vi "receiveBLMessages.vi"(8 "Error in":errorcluster {"code" format="%.0x"}, 11 "ObjHandle in":T2) -> (0 "Error out":errorcluster {"code" format="%.0x"}, 1 "msgData":T1[](array[typedef]) {"Data" format="%.0x"; "ArbitrationId" format="%.0x"; "Timestamp" format="%<%I:%M:%S%3u %p\n%m/%d/%Y>T"}, 2 "msgCount":u32, 3 "ObjHandle out":T2, 6 "msgIDs":u32[](array[numeric]) format="%.0x")   [LabVIEW 2017]
uses:
  <vilib>/nican/nican.llb/xobjhandle.ctl
  <vilib>/nican/nican.llb/CanFrameTimed.ctl
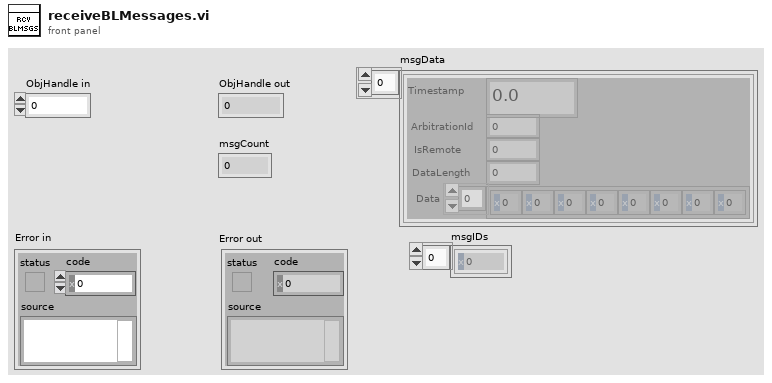
[diagram p1: front panel]
types:
  T1 = typedef "CanFrameTimed.ctl" = cluster{"Timestamp":dbl, "ArbitrationId":u32, "IsRemote":u8, "DataLength":u8, "Data":u8[]}
  T2 = typedef "xobjhandle.ctl" = u32
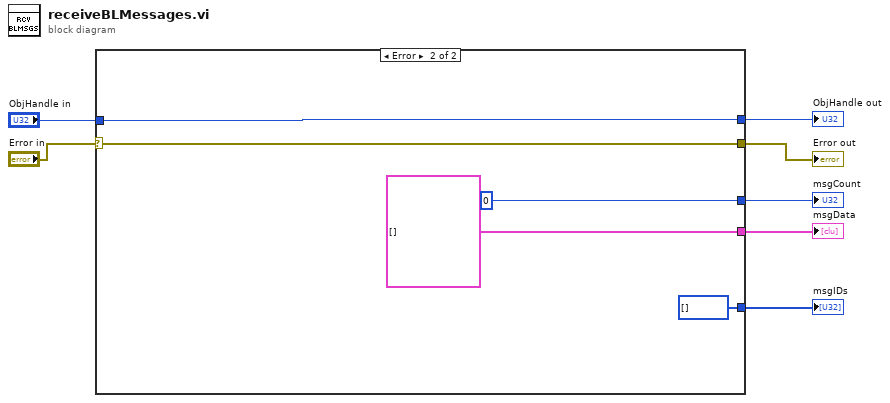
[diagram p0: block diagram]
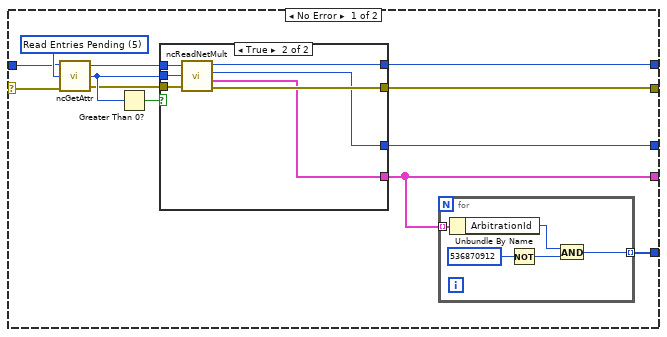
[diagram p2: hidden frame]
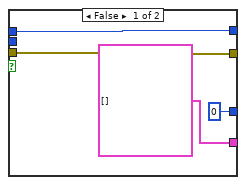
[diagram p3: hidden frame]
diagram:
  n1 = case shown="Error" "Error in" {
    selector: "Error in" -> [w11 w39]
    tunnel: "ObjHandle in" -> [w12 w40]
    tunnel: [w14 w40] -> w6
    tunnel: [w10 w39] -> w4
    tunnel: [w9 T1[] [] ("Data")] -> w3
    tunnel: [w13 u32 0 ("ActualDataSize (Frames)")] -> w2
    tunnel: [w8 u32[] []] -> w1
    frame No Error {
      w15 = u32 5 items=["(reserved)", "Protocol Version", "Software Version", "Object State", "(reserved)", "Read Entries Pending", "Write Entries Pending", "ReadMult Size for Notification", "Listen Only?", "Self Reception?", "Transmit Error Counter", "Receive Error Counter", "Single Shot Transmit?", "Series 2 Filter Mode", "Series 2 Mask", "Series 2 Comparator", "Serial Number", "Form Factor", "Series", "Transceiver Type", "Interface Number", "Series 2 Error/Arb Capture", "Transceiver Mode", "Transceiver External Outputs", "Transceiver External Inputs", "Start Trigger Behavior", "Log Comm Warnings", "User RTSI Frame", "Transmit Mode", "Log Start Trigger?", "Timestamp Format", "Master Timebase Rate", "Virtual Bus Timing"] ("AttrId")
      n2 = call <vilib>:"ncGetAttr.vi"("Error in"=w11, "AttrId"=w15, "ObjHandle in"=w12) -> ("Error out"=w16:errorcluster, "AttrValue"=w19:u32, "ObjHandle out"=w17:T2)
      n3 = Greater Than 0?(x=w19) -> (x > 0?=w18:bool)
      n4 = case shown="True" w18 {
        tunnel: [w27 w35] -> w10
        tunnel: [w28 w34] -> w14
        tunnel: w19 -> [_ w33]
        tunnel: w16 -> [w27 w32]
        tunnel: w17 -> [w28 w31]
        tunnel: [T1[] [] ("Data") w30] -> w9
        tunnel: [u32 0 ("ActualDataSize (Frames)") w29] -> w13
        frame False {
        }
        frame True {
          n5 = call <vilib>:"ncReadNetMult.vi"("ObjHandle in"=w31, "Requested Number of Frames"=w33, "Error in"=w32) -> ("ObjHandle out"=w34:T2, "ActualDataSize (Frames)"=w29:u32, "Data"=w30:T1[], "Error out"=w35:errorcluster)
        }
      }
      n6 = for {
        tunnel: w9 -> [w24] mode=indexing
        tunnel: [w20] -> w8 mode=indexing
        n7 = Unbundle By Name(w24) -> ("ArbitrationId"=w22:u32)
        n8 = Not(x=u32 536870912 ("y")) -> (.not. x?=w21:u32)
        n9 = And(x=w22, y=w21) -> (x .and. y?=w20:u32)
      }
    }
    frame Error {
    }
  }
  "ObjHandle out" <- w6
  "Error out" <- w4
  "msgData" <- w3
  "msgCount" <- w2
  "msgIDs" <- w1
